vi "Move to (SubVI).vi"(10 "字符串":string, 11 ".NET引用句柄输入":refnum<k24>) -> (0 "错误输出":errorcluster)   [LabVIEW 2019, in "SubVI.lvlib"]
uses:
  SubVI.lvlib
  lib/QDInstrument.dll
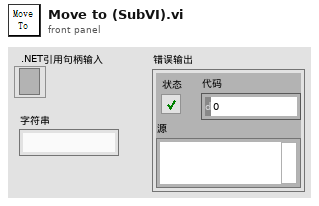
[diagram p1: front panel]
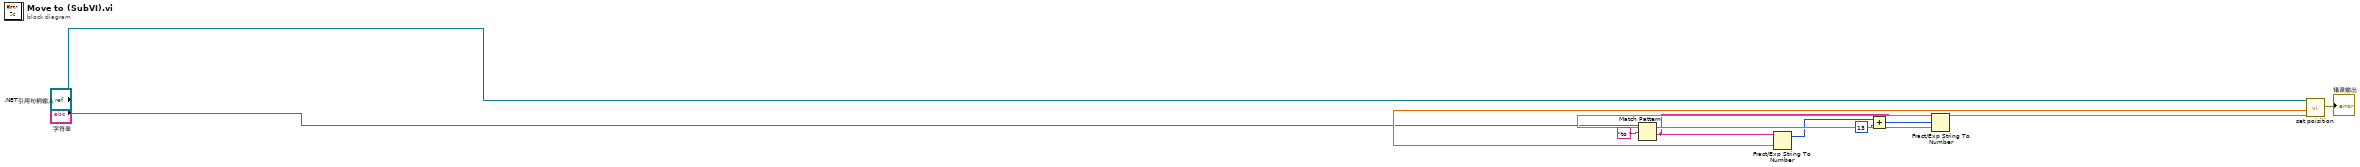
[diagram p0: block diagram]
diagram:
  n1 = Match Pattern(string="字符串", regular expression="to " ("正则表达式")) -> (after substring=w7:string)  [unwired: 1 in, 3 out]
  n2 = Fract/Exp String To Number(string=w7) -> (offset past number=w5:i32, number=w3:dbl)  [unwired: 3 in]
  n3 = Add(x=w5, y=13) -> (x+y=w8:i32)
  n4 = Fract/Exp String To Number(string=w7, offset=w8) -> (number=w9:dbl)  [unwired: 2 in, 1 out]
  n5 = call "set poisition.vi"("Slow down code\ndefault = 0"=w9, "Position (deg)"=w3, "Instrument Ref In"=".NET引用句柄输入") -> ("error out"=→"错误输出":errorcluster)  [unwired: 5 in, 1 out]
